vi "Estructura de control Case.vi"() -> ()   [LabVIEW 2015]
panel:
  out "Resultado":dbl
  in  "Numero B":dbl
  in  "Numero A":dbl
  in  "Decision":dbl
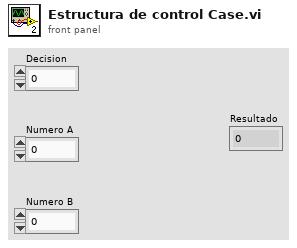
[diagram p1: front panel]
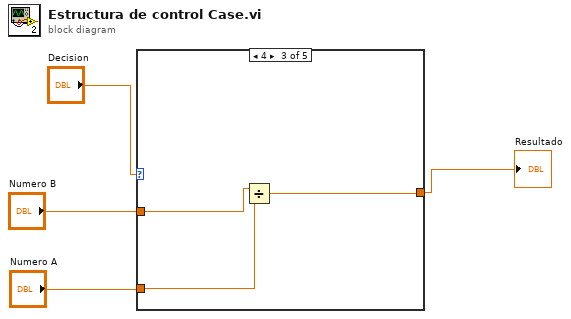
[diagram p0: block diagram]
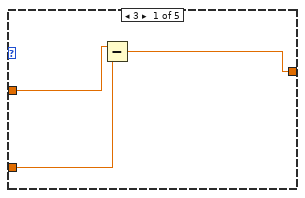
[diagram p2: hidden frame]
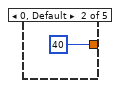
[diagram p3: hidden frame]
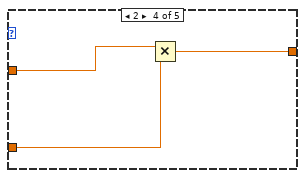
[diagram p4: hidden frame]
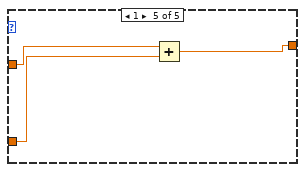
[diagram p5: hidden frame]
diagram:
  n1 = case shown="4" "Decision" {
    tunnel: "Numero B" -> [w7 _ w11 w14 w17]
    tunnel: "Numero A" -> [w6 _ w10 w13 w16]
    tunnel: [w5 40 w9 w12 w15] -> w4
    frame 3 {
      n2 = Subtract(x=w7, y=w6) -> (x-y=w5:dbl)
    }
    frame 0, Default {
    }
    frame 4 {
      n3 = Divide(x=w11, y=w10) -> (x/y=w9:dbl)
    }
    frame 2 {
      n4 = Multiply(x=w14, y=w13) -> (x*y=w12:dbl)
    }
    frame 1 {
      n5 = Add(x=w17, y=w16) -> (x+y=w15:dbl)
    }
  }
  "Resultado" <- w4
